vi "String Indent Code.vi"(10 "complete code":string, 11 "actual nested level":i32) -> (3 "indented code":string)   [LabVIEW 2014]
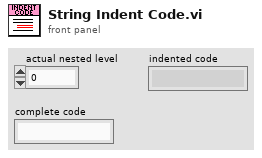
[diagram p1: front panel]
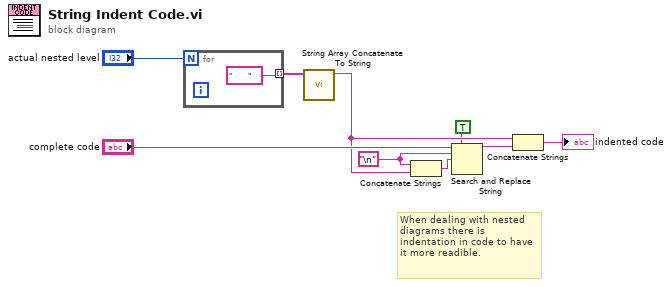
[diagram p0: block diagram]
diagram:
  w8 = "\n" ("Line Feed Constant")
  # "When dealing with nested diagrams there is indentation in code to have it more readible."
  n1 = for {
    N: "actual nested level" -> [_]
    tunnel: ["        " ("string")] -> w6 mode=indexing
  }
  n2 = call "String Array Concatenate To String.vi"("Array String In"=w6) -> ("String"=w7:string)  [unwired: 10 in]
  n3 = Concatenate Strings(w8, w7) -> (w2:string)
  n4 = Search and Replace String(replace all?=TRUE ("replace all? (F)"), input string="complete code", search string=w8, replace string=w2) -> (result string=w3:string)  [unwired: 4 in, 3 out]
  n5 = Concatenate Strings(w7, w3) -> (→"indented code":string)
